vi "handle_connection.vi"(6 "Log Service":refnum<data-value>, 8 "error in (no error)":errorcluster, 10 "connection":refnum<class "Connection.lvclass">, 11 "Enumerating Connection Handler in":refnum<class "Enumerating Connection Handler.lvclass">) -> (0 "error out":errorcluster)   [LabVIEW 2019, in "Enumerating Connection Handler.lvclass"]
uses:
  Enumerating Connection Handler.lvclass
  Connection/Connection.lvclass
  Utility API/Log Service/Log Service.lvclass
  Enumerating Connection Handler.lvclass/Enumerating Connection Handler.ctl
  Utility API/Log Service/public/level.ctl
  27740510-d790-4795-b017-20472e36913b.vi
  8ee5640b-7bbc-4240-ad00-c674961e8a8e.vi
  Util/Timestamp or now.vi
  Connection Handler/Connection Handler.lvclass
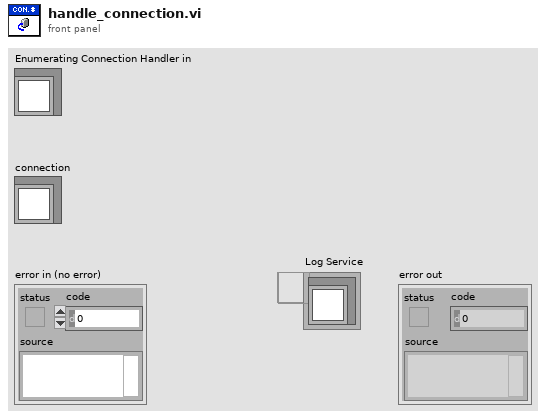
[diagram p1: front panel]
types:
  T1 = typedef "Utility API.lvlib/Log Service.lvclass/level.ctl" = u16
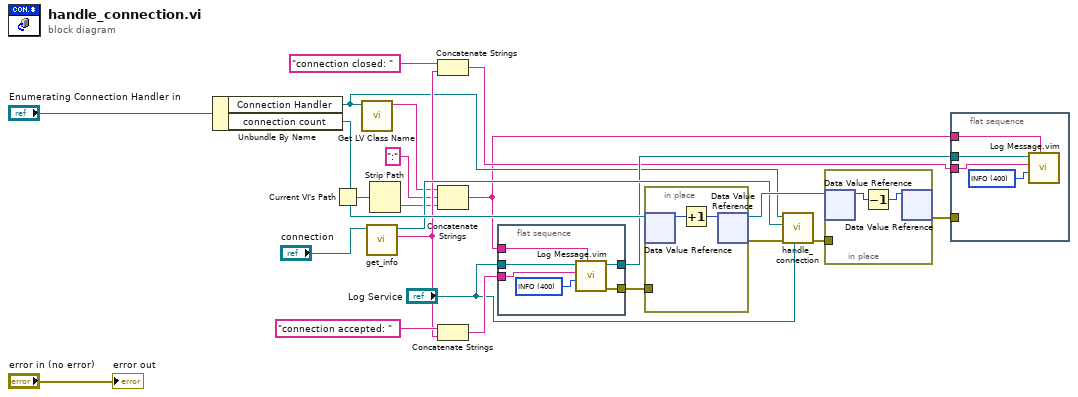
[diagram p0: block diagram]
diagram:
  n1 = Unbundle By Name("Enumerating Connection Handler in") -> ("Connection Handler"=w5:refnum<class "Connection Handler.lvclass">, "connection count"=w21:refnum<data-value>)
  n2 = Current VI's Path() -> (path=w17:path)
  n3 = call <vilib>:"Get LV Class Name.vi"("object"=w5) -> ("class name"=w3:string)  [unwired: 9 in, 1 out]
  n4 = call-dynamic "get_info.vi"("Connection in"="connection") -> ("info."=w10:string, "Connection out"=w15:refnum<class "Connection.lvclass">)  [unwired: 8 in, 1 out]
  n5 = Strip Path(path=w17) -> (name=w2:string)  [unwired: 1 out]
  n6 = Concatenate Strings("connection closed: ", w10) -> (w9:string)
  n7 = Concatenate Strings(w3, ":" ("string"), w2) -> (w1:string)
  n8 = Concatenate Strings("connection accepted: ", w10) -> (w13:string)
  n9 = flat-sequence {
    tunnel: "Log Service" -> [w29]
    tunnel: w13 -> [w28]
    tunnel: [w27] -> w12
    tunnel: w1 -> [w26]
    tunnel: [w24] -> w8
    frame #0 {
      w25 = T1 400 items=["OFF"=0, "FATAL"=100, "ERROR"=200, "WARN"=300, "INFO"=400, "DEBUG"=500, "TRACE"=600, "ALL"=65535] ("level")
      n10 = call "Log Message.vim"("context"=w26, "level"=w25, "message"=w28, "Log Service in"=w29) -> ("error out"=w24:errorcluster, "Log Service out"=w27:refnum<data-value>)  [unwired: 6 in]
    }
  }
  n11 = in-place {
    in-place-border: w8 -> [_]
    n12 = in-place-dvr #1(w21) -> (w31:i32)  [unwired: 1 out]
    n13 = Increment(x=w31) -> (x+1=w30:i32)
    n14 = in-place-dvr #1(w30) -> (w18:refnum<data-value>, w20:errorcluster)
  }
  n15 = call-dynamic "handle_connection.vi"("Log Service"="Log Service", "error in (no error)"=w20, "connection"=w15, "Connection Handler in"=w5) -> ("error out"=w19:errorcluster)  [unwired: 7 in]
  n16 = in-place {
    in-place-border: w19 -> [_]
    n17 = in-place-dvr #2(w18) -> (w33:i32)  [unwired: 1 out]
    n18 = Decrement(x=w33) -> (x-1=w32:i32)
    n19 = in-place-dvr #2(w32) -> (w7:errorcluster)  [unwired: 1 out]
  }
  n20 = flat-sequence {
    tunnel: w12 -> [w37]
    tunnel: w1 -> [w36]
    tunnel: w9 -> [w35]
    tunnel: w7 -> [_]
    frame #0 {
      w34 = T1 400 items=["OFF"=0, "FATAL"=100, "ERROR"=200, "WARN"=300, "INFO"=400, "DEBUG"=500, "TRACE"=600, "ALL"=65535] ("level")
      n21 = call "Log Message.vim"("context"=w36, "level"=w34, "message"=w35, "Log Service in"=w37) -> ()  [unwired: 6 in, 2 out]
    }
  }
  "error out" <- "error in (no error)"
